vi "fakeScan.vi"() -> ()   [LabVIEW 2010]
panel:
  in  "volume info":T1
  in  "fake 2 ch im":u32[](array[numeric])
  in  "scan specification":T2={"x amplitude"=100, "x resolution (pixels)"=28, "x offset fly-forward (iterations)"=50, "x offset fly-back (iterations)"=100, "y resolution (nr. of lines)"=80, "y step size"=30, "iterations per pixel"=5, "number of frames"=80, "y offset (pixels)"=0, "number of y-brake lines  (before y-fly-back)"=0, "number y-brake lines (after y-fly-back)"=40, "number of y-fly-back steps"=0, "lines per z step"=1, "number of z/intensity tuples"=228, "number of repetitions (volumes or planes)"=1000, "z step size derived"=32, "choose the beginning of z scan"=FALSE, "number of frames (settings)"=80, "FPGA trajectory?"=TRUE, "Pockels cell voltage (bits)"=0, "Vy min(bits)"=0, "Vz min(bits)"=0}
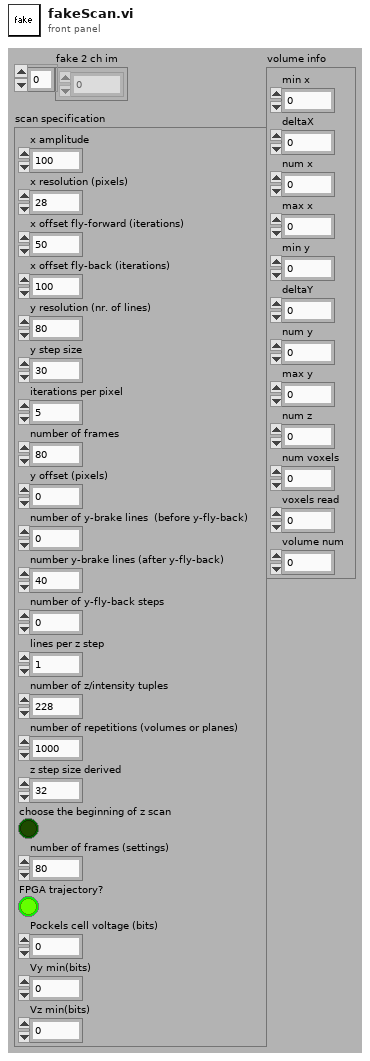
[diagram p1: front panel]
types:
  T1 = cluster{"min x":i16, "deltaX":dbl, "num x":u32, "max x":i16, "min y":i16, "deltaY":dbl, "num y":u32, "max y":i16, "num z":u32, "num voxels":u32, "voxels read":u32, "volume num":u32}
  T2 = cluster{"x amplitude":u16, "x resolution (pixels)":u16, "x offset fly-forward (iterations)":u16, "x offset fly-back (iterations)":u16, "y resolution (nr. of lines)":u16, "y step size":u16, "iterations per pixel":u16, "number of frames":i32, "y offset (pixels)":u16, "number of y-brake lines  (before y-fly-back)":u16, "number y-brake lines (after y-fly-back)":u16, "number of y-fly-back steps":u16, "lines per z step":u16, "number of z/intensity tuples":u16, "number of repetitions (volumes or planes)":i32, "z step size derived":u16, "choose the beginning of z scan":bool, "number of frames (settings)":i32, "FPGA trajectory?":bool, "Pockels cell voltage (bits)":i16, "Vy min(bits)":i16, "Vz min(bits)":i16}
  T3 = cluster{"volumeQueue":refnum<queue>, "lineQueue":refnum<queue>, "comQueue":refnum<queue>, "completedVolumeQueue":refnum<queue>, "displayVolumeQueue":refnum<queue>}
  T4 = cluster{"start X":i16, "start Y":i16, "start Z":i16, "end X":i16, "end Y":i16, "end Z":i16, "num z":u8, "voxel data":u32[], "volume num":u32}
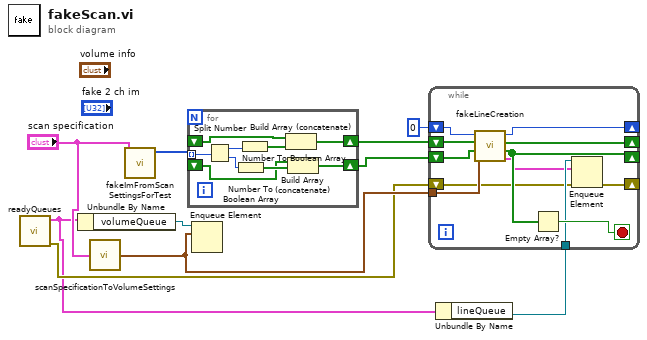
[diagram p0: block diagram]
diagram:
  n1 = call "readyQueues.vi"() -> ("error out"=w2:errorcluster, "Queues"=w1:T3)  [unwired: 10 in]
  n2 = Unbundle By Name(w1) -> ("volumeQueue"=w10:refnum<queue>)
  n3 = call "scanSpecificationToVolumeSettings.vi"("scan specification"="scan specification") -> ("volume info"=w5:T1)
  n4 = call "fakeImFromScanSettingsForTest.vi"("scan specification"="scan specification") -> ("fake 2 ch im"=w8:u32[])  [unwired: 10 in]
  n5 = for {
    tunnel: w8 -> [w19] mode=indexing
    shift-right: [w14] -> w6
    shift-left: _ -> [w13]
    shift-right: [w12] -> w7
    shift-left: _ -> [w11]
    n6 = Split Number(x=w19) -> (hi(x)=w18:u16, lo(x)=w17:u16)
    n7 = Number To Boolean Array(number=w17) -> (Boolean array=w16:bool[])
    n8 = Number To Boolean Array(number=w18) -> (Boolean array=w15:bool[])
    n9 = Build Array (concatenate)(w11, w15) -> (w12:bool[])
    n10 = Build Array (concatenate)(w13, w16) -> (w14:bool[])
  }
  n11 = Enqueue Element(queue=w10, element=w5) -> ()  [unwired: 2 in, 3 out]
  n12 = Unbundle By Name(w1) -> ("lineQueue"=w3:refnum<queue>)
  n13 = while {
    tunnel: w5 -> [w29]
    shift-right: [w27] -> _
    shift-left: w6 -> [w30]
    shift-right: [w26] -> _
    shift-left: w7 -> [w31]
    shift-right: [w25] -> _
    shift-left: u32 0 ("voxel number out") -> [w24]
    tunnel: w3 -> [w23]
    shift-right: [w21] -> _
    shift-left: w2 -> [w20]
    stop <- w28 stop-if-true
    n14 = call "fakeLineCreation.vi"("volume info"=w29, "ch1"=w30, "ch0"=w31, "voxel number"=w24) -> ("line"=w22:T4, "ch1 out"=w27:bool[], "ch0 out"=w26:bool[], "voxel number out"=w25:u32)  [unwired: 4 in]
    n15 = Empty Array?(array=w27) -> (empty?=w28:bool)
    n16 = Enqueue Element(queue=w23, element=w22, error in (no error)=w20) -> (error out=w21:errorcluster)  [unwired: 1 in, 2 out]
  }
